vi "HexapodAcquireHardware.vi"(8 "error in (no error)":errorcluster, 11 "HexapodPI in":refnum<class "HexapodPI.lvclass">) -> (0 "error out":errorcluster, 1 "Status Cluster":T1, 2 "In Motion":bool, 3 "HexapodPI out":refnum<class "HexapodPI.lvclass">, 5 "Array":string[](array[string]))   [LabVIEW 2020, in "HexapodPI.lvclass"]
uses:
  HexapodPI.lvclass
  HexapodPI.lvclass/HexapodPI.ctl
  subvis/activeChannel.ctl
  shared/OnOffTypeDef.ctl
  shared/CompressAndUpdate(Poly)/CompressAndUpdate(Enum).vi
  shared/CompressAndUpdate(Poly)/CompressAndUpdate(Numeric).vi
  shared/CompressAndUpdate(Poly)/CompressAndUpdate(NumericArray).vi
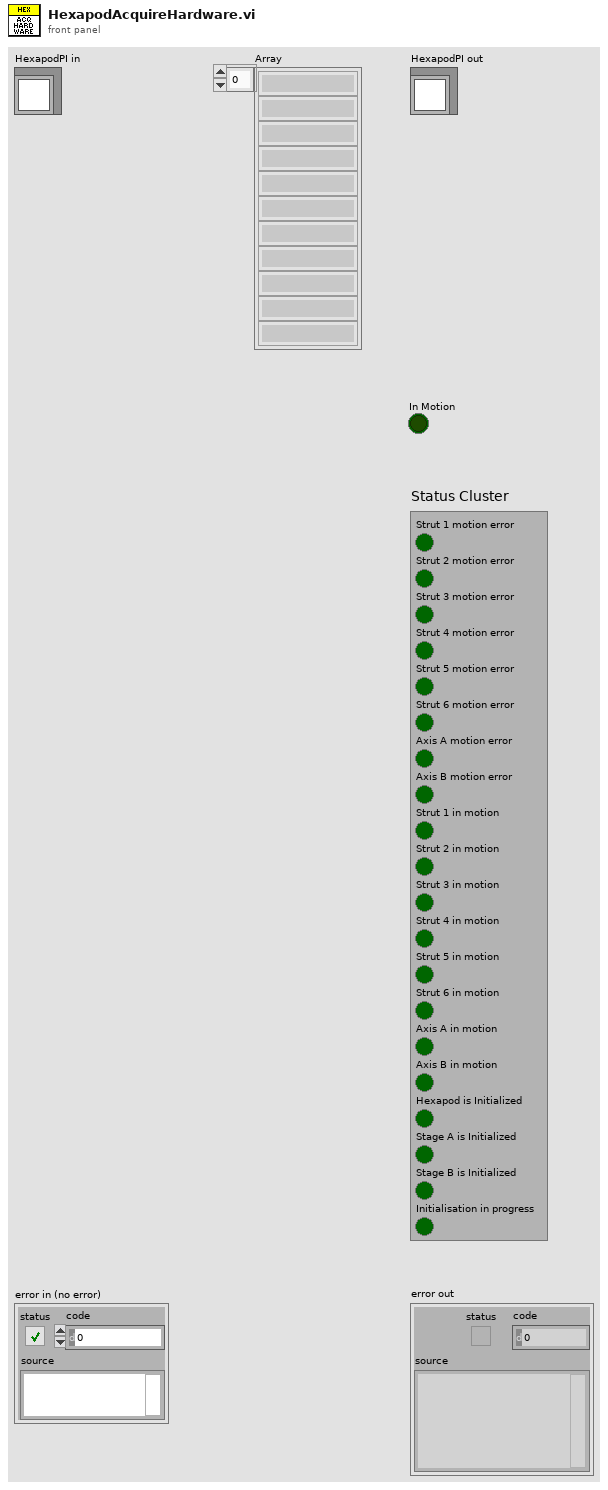
[diagram p1: front panel]
types:
  T1 = cluster{"Strut 1 motion error":bool, "Strut 2 motion error":bool, "Strut 3 motion error":bool, "Strut 4 motion error":bool, "Strut 5 motion error":bool, "Strut 6 motion error":bool, "Axis A motion error":bool, "Axis B motion error":bool, "Strut 1 in motion":bool, "Strut 2 in motion":bool, "Strut 3 in motion":bool, "Strut 4 in motion":bool, "Strut 5 in motion":bool, "Strut 6 in motion":bool, "Axis A in motion":bool, "Axis B in motion":bool, "Hexapod is Initialized":bool, "Stage A is Initialized":bool, "Stage B is Initialized":bool, "Initialisation in progress":bool}
  T2 = enum16{"Not referenced", "Homing", "Moving", "Ready"}
  T3 = typedef "activeChannel.ctl" = enum16{"xpos", "ypos", "zpos", "uangle", "vangle", "wangle", "n/a", "off"}
  T4 = typedef "OnOffTypeDef.ctl" = enum16{"off", "on"}
  T5 = cluster{"Zpos":T4, "Zneg":T4, "Xpos":T4, "Xneg":T4, "Ypos":T4, "Yneg":T4, "Wpos":T4, "Wneg":T4, "Vpos":T4, "Vneg":T4, "Upos":T4, "Uneg":T4}
  T6 = cluster{"connection ID":refnum<k5>, "VISA resource name":refnum<visa-resource-name>, "Selector":enum16{"TCPIP", "Serial"}}
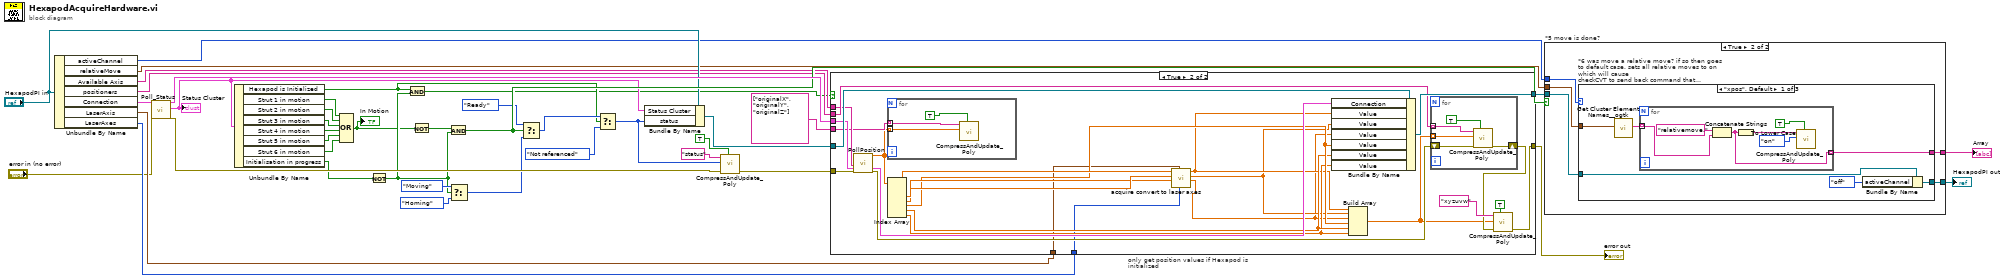
[diagram p0: block diagram]
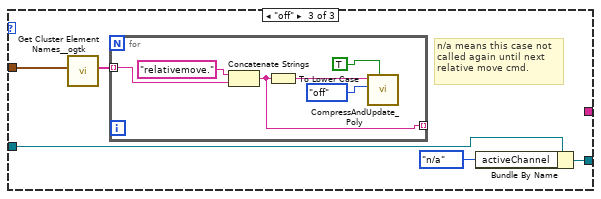
[diagram p4: hidden frame]
diagram:
  n1 = Unbundle By Name("HexapodPI in") -> ("activeChannel"=w2:T3, "relativeMove"=w33:T5, "Available Axis"=w30:string[], "positioners"=w29:string[], "Connection"=w4:T6, "LaserAxis"=w39:cluster{"u":dbl, "v":dbl, "w":dbl}, "LaserAxes"=w41:T4)
  n2 = call "Poll_Status.vi"("Connection"=w4, "error in"="error in (no error)") -> ("Connection out"=w40:T6, "Status Cluster"=w31:T1, "error out"=w24:errorcluster)  [unwired: 15 in]
  "Status Cluster" <- w31
  n3 = Unbundle By Name(w31) -> ("Hexapod is Initialized"=w21:bool, "Strut 1 in motion"=w12:bool, "Strut 2 in motion"=w7:bool, "Strut 3 in motion"=w8:bool, "Strut 4 in motion"=w9:bool, "Strut 5 in motion"=w10:bool, "Strut 6 in motion"=w11:bool, "Initialisation in progress"=w6:bool)
  n4 = Compound Arithmetic op=OR(w12, w7, w8, w9, w10, w11) -> (w16:bool)
  "In Motion" <- w16
  n5 = Not(x=w6) -> (.not. x?=w17:bool)
  n6 = And(x=w21, y=w17) -> (x .and. y?=w13:bool)
  n7 = Not(x=w16) -> (.not. x?=w32:bool)
  n8 = And(x=w32, y=w17) -> (x .and. y?=w37:bool)
  n9 = Select(t=T2."Moving" ("Settings.status"), s=w17, f=T2."Homing" ("Settings.status")) -> (s? t:f=w18:T2)
  n10 = Select(t=T2."Ready" ("Settings.status"), s=w37, f=w18) -> (s? t:f=w22:T2)
  n11 = Select(t=w22, s=w21, f=T2."Not referenced" ("Settings.status")) -> (s? t:f=w26:T2)
  n12 = Bundle By Name(cluster="HexapodPI in", "Status Cluster"=w31, "status"=w26) -> (w14:refnum<class "HexapodPI.lvclass">)
  n13 = call-poly "CompressAndUpdate_Poly.vi"("force CVT update (false)"=TRUE, "error in"=w24, "enum variant"=w26, "command or variable name"="status") -> ("error out"=w25:errorcluster)  [unwired: 7 in]
  n14 = case "only get position values if Hexapod is initialized" shown="True" w13 {
    tunnel: [w42 w45] -> w1
    tunnel: [w43 w69] -> w35
    tunnel: w14 -> [w43 w68]
    tunnel: w25 -> [w42 w67]
    tunnel: w40 -> [_ w66]
    tunnel: w29 -> [_ w63]
    tunnel: w30 -> [_ w62]
    tunnel: string[] ["originalX", "originalY", "originalZ"] -> [_ w55]
    tunnel: w39 -> [_ w50]
    tunnel: w41 -> [_ w49]
    frame False {
    }
    frame True {
      n15 = call "PollPosition.vi"("Queried axes"=w62, "Connection"=w66, "error in"=w67) -> ("Position"=w54:dbl[], "Connection out"=w64:T6, "error out"=w65:errorcluster)  [unwired: 13 in, 1 out]
      n16 = for {
        tunnel: w54 -> [w71] mode=indexing
        tunnel: w55 -> [w70] mode=indexing
        n17 = call-poly "CompressAndUpdate_Poly.vi"("force CVT update (false)"=TRUE, "Numeric"=w71, "command or variable name"=w70) -> ()  [unwired: 8 in, 1 out]
      }
      n18 = Index Array(array=w54) -> (element #1=w61:dbl, element #2=w60:dbl, element #3=w59:dbl, element #4=w58:dbl, element #5=w57:dbl, element #6=w56:dbl)  [unwired: 6 in]
      n19 = call "acquire convert to laser axes.vi"("Settings.Trigger"=w49, "LaserAxis"=w50, "z in"=w59, "y in"=w60, "x in"=w61) -> ("z out"=w51:dbl, "y out"=w52:dbl, "x out"=w53:dbl)  [unwired: 4 in]
      n20 = Bundle By Name(cluster=w68, "Connection"=w64, "Value"=w53, "Value"=w52, "Value"=w51, "Value"=w58, "Value"=w57, "Value"=w56) -> (w69:refnum<class "HexapodPI.lvclass">)
      n21 = Build Array(w53, w52, w51, w58, w57, w56) -> (w44:dbl[])
      n22 = for {
        tunnel: w44 -> [w74] mode=indexing
        tunnel: w63 -> [w73] mode=indexing
        shift-right: [w77] -> w46
        shift-left: w65 -> [w75]
        n23 = call-poly "CompressAndUpdate_Poly.vi"("force CVT update (false)"=TRUE, "error in"=w75, "Numeric"=w74, "command or variable name"=w73) -> ("error out"=w77:errorcluster)  [unwired: 7 in]
      }
      n24 = call-poly "CompressAndUpdate_Poly.vi"("force CVT update (false)"=TRUE, "error in"=w46, "Numeric Array"=w44, "command or variable name"="xyzuvw") -> ("error out"=w45:errorcluster)  [unwired: 7 in]
    }
  }
  "error out" <- w1
  n25 = case "*5 move is done?" shown="True" w37 {
    tunnel: w33 -> [_ w83]
    tunnel: w2 -> [_ w82]
    tunnel: w35 -> [w78 w81]
    tunnel: [w78 w80] -> w36
    tunnel: [_ w79] -> w3
    frame False {
    }
    frame True {
      n26 = case "*6 was move a relative move? if so then goes to default case. sets all relative moves to on which will cause\ncheckCVT to send back command that setrelative move was done. sets activechannel to off so next acquire will\nset all relative move enums to off." shown="\"xpos\", Default" w82 {
        tunnel: w83 -> [w89 _ w100]
        tunnel: w81 -> [w88 w96 w99]
        tunnel: [w87 w96 w97] -> w80
        tunnel: [w84 _ _] -> w79
        frame "xpos", Default {
          n27 = call <userlib>:"Get Cluster Element Names__ogtk.vi"("Cluster"=w89) -> ("Element Names"=w86:string[])  [unwired: 9 in, 1 out]
          n28 = for {
            tunnel: w86 -> [w95] mode=indexing
            tunnel: [w91] -> w84 mode=indexing
            n29 = Concatenate Strings("relativemove." ("string"), w95) -> (w91:string)
            n30 = To Lower Case(string=w91) -> (all lower case string=w90:string)
            n31 = call-poly "CompressAndUpdate_Poly.vi"("force CVT update (false)"=TRUE, "enum variant"=OnOffTypeDef."on" ("Zpos"), "command or variable name"=w90) -> ()  [unwired: 8 in, 1 out]
          }
          n32 = Bundle By Name(cluster=w88, "activeChannel"=activeChannel."off") -> (w87:refnum<class "HexapodPI.lvclass">)
        }
        frame "n/a" {
        }
        frame "off" {
          # "n/a means this case not\ncalled again until next\nrelative move cmd."
          n33 = call <userlib>:"Get Cluster Element Names__ogtk.vi"("Cluster"=w100) -> ("Element Names"=w101:string[])  [unwired: 9 in, 1 out]
          n34 = for {
            tunnel: w101 -> [w107] mode=indexing
            tunnel: [w103] -> _ mode=indexing
            n35 = Concatenate Strings("relativemove." ("string"), w107) -> (w103:string)
            n36 = To Lower Case(string=w103) -> (all lower case string=w102:string)
            n37 = call-poly "CompressAndUpdate_Poly.vi"("force CVT update (false)"=TRUE, "enum variant"=OnOffTypeDef."off" ("Zpos"), "command or variable name"=w102) -> ()  [unwired: 8 in, 1 out]
          }
          n38 = Bundle By Name(cluster=w99, "activeChannel"=activeChannel."n/a") -> (w97:refnum<class "HexapodPI.lvclass">)
        }
      }
    }
  }
  "HexapodPI out" <- w36
  "Array" <- w3
